vi "generate_tuning_spline.vi"(0 "Laser Power Q":T3, 11 "error in":errorcluster, 12 "Controls Cluster":T2 {"Initial Step Direction" items=["Negative", "Positive"]}, 13 "file path (dialog if empty)":path, 14 "Bounds":T1) -> (4 "Opt Data":cluster{dbl[], dbl[]}, 15 "error out":errorcluster)   [LabVIEW 2023]
uses:
  <vilib>/Utility/file.llb/Write Delimited Spreadsheet (DBL).vi
panel:
  in  "Cancel Optimisation":bool
  in  "stop":bool
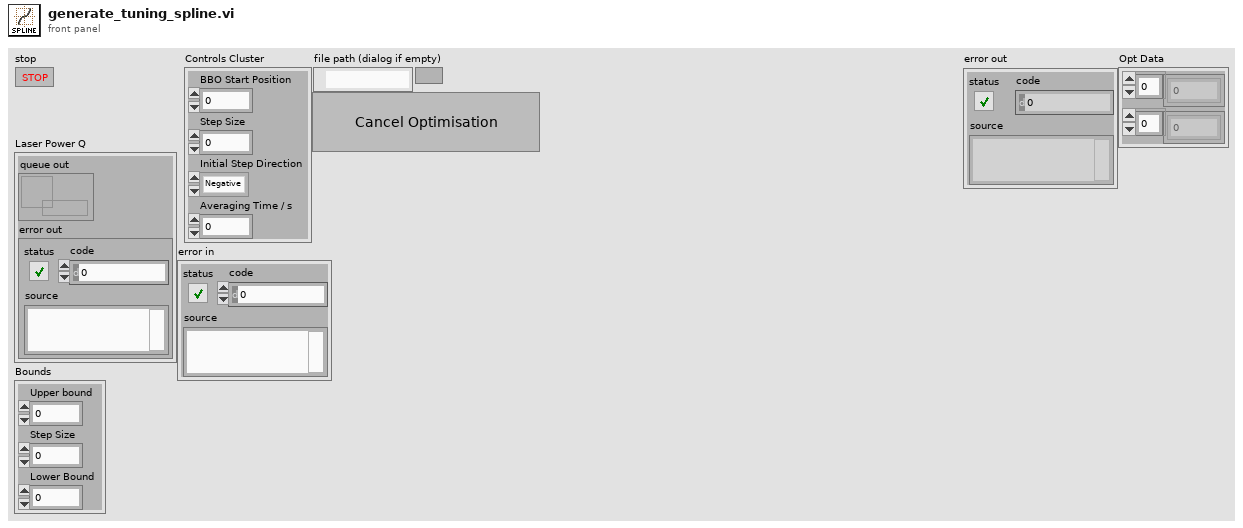
[diagram p1: front panel]
types:
  T1 = cluster{"Upper bound":dbl, "Step Size":dbl, "Lower Bound":dbl}
  T2 = cluster{"BBO Start Position":i32, "Step Size":i32, "Initial Step Direction":u16, "Averaging Time / s ":u32}
  T3 = cluster{"queue out":refnum<queue>, "error out":errorcluster}
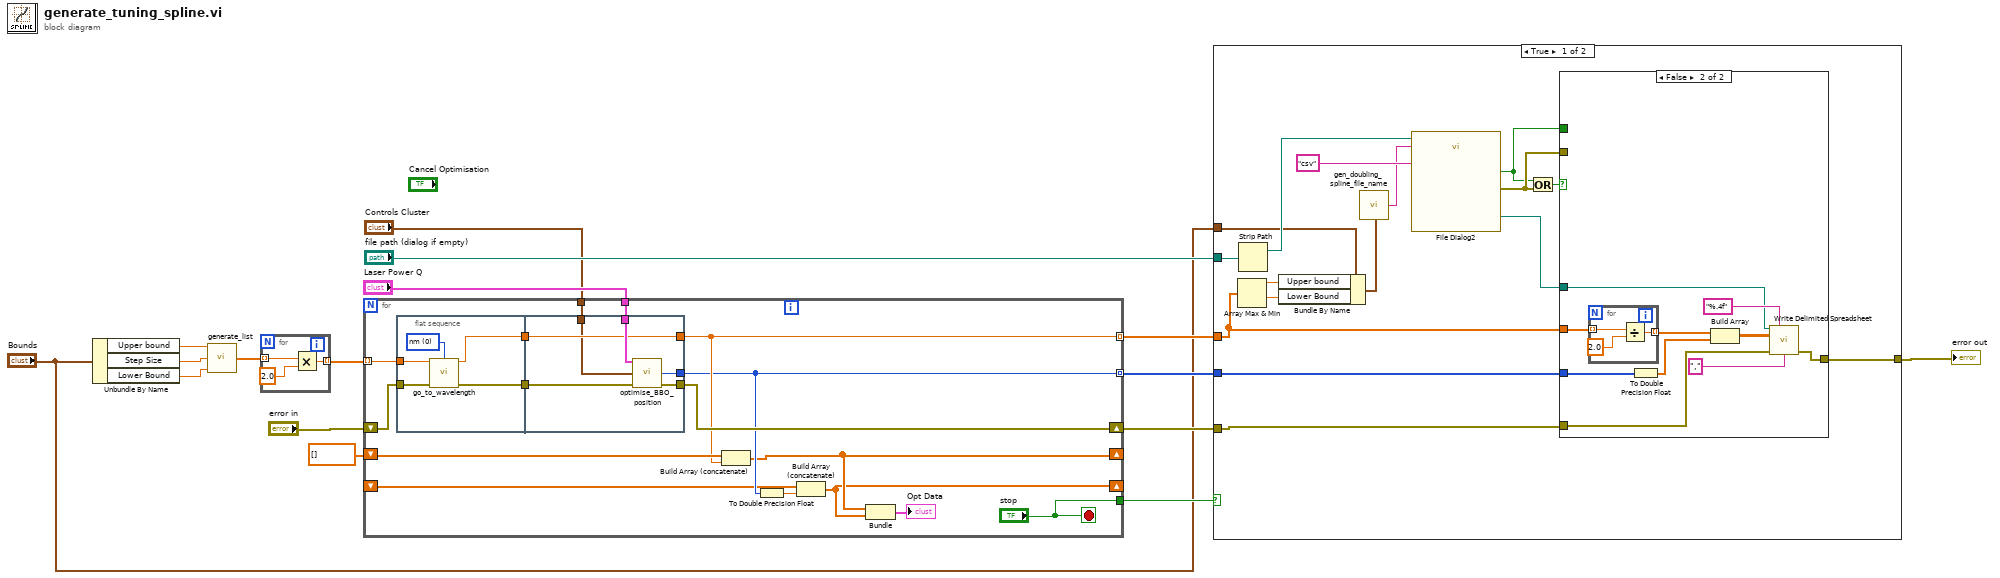
[diagram p0: block diagram]
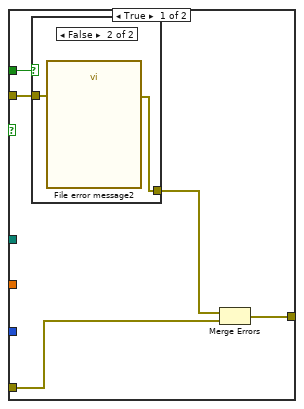
[diagram p2: hidden frame]
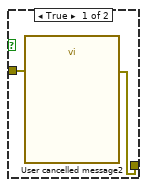
[diagram p3: hidden frame]
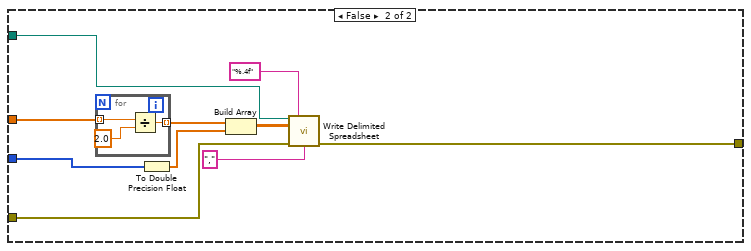
[diagram p4: hidden frame]
diagram:
  n1 = Unbundle By Name("Bounds") -> ("Upper bound"=w8:dbl, "Step Size"=w7:dbl, "Lower Bound"=w6:dbl)
  n2 = call "generate_list.vi"("Upper bound"=w8, "Step Size"=w7, "Lower Bound"=w6) -> ("Array"=w16:dbl[])  [unwired: 12 in]
  n3 = for {
    tunnel: w16 -> [w19] mode=indexing
    tunnel: [w17] -> w15 mode=indexing
    n4 = Multiply(x=w19, y=2.0) -> (x*y=w17:dbl)
  }
  n5 = for {
    tunnel: w15 -> [w35] mode=indexing
    shift-right: [w32] -> w10
    shift-left: "error in" -> [w34]
    tunnel: "Laser Power Q" -> [w31]
    tunnel: [w27] -> w11 mode=indexing
    tunnel: [w28] -> w12 mode=indexing
    shift-right: [w24] -> _
    shift-left: dbl[] [] -> [w29]
    shift-right: [w23] -> _
    shift-left: _ -> [w25]
    tunnel: "Controls Cluster" -> [w21]
    tunnel: ["stop"] -> w4
    stop <- "stop" stop-if-true
    n6 = flat-sequence {
      tunnel: w35 -> [w40]
      tunnel: w34 -> [w39]
      tunnel: [w37] -> w33
      tunnel: [w36] -> w30
      tunnel: [w44] -> w32
      tunnel: w33 -> [w46]
      tunnel: w31 -> [w45]
      tunnel: [w43] -> w27
      tunnel: w30 -> [w42]
      tunnel: [w42] -> w28
      tunnel: w21 -> [w41]
      frame #0 {
        w38 = u16 0 items=["nm", "cm-1"] ("Unit")
        n7 = call "go_to_wavelength.vi"("Set Laser Position"=w40, "Unit"=w38, "error in (no error)"=w39) -> ("Current Laser Position"=w36:dbl, "error out"=w37:errorcluster)  [unwired: 11 in]
      }
      frame #1 {
        n8 = call "optimise_BBO_position.vi"("Laser Power Q"=w45, "Controls Cluster"=w41, "error in (no error)"=w46) -> ("Optimised BBO crystal position"=w43:i32, "error out"=w44:errorcluster)  [unwired: 11 in]
      }
    }
    n9 = Build Array (concatenate)(w29, w28) -> (w24:dbl[])
    n10 = To Double Precision Float(number=w27) -> (double precision float=w26:dbl)
    n11 = Build Array (concatenate)(w25, w26) -> (w23:dbl[])
    n12 = Bundle(w24, w23) -> (→"Opt Data":cluster{dbl[], dbl[]})  [unwired: 1 in]
  }
  n13 = case shown="True" w4 {
    tunnel: w12 -> [w53 w94]
    tunnel: w11 -> [w56 w93]
    tunnel: w10 -> [w57 w89]
    tunnel: "file path (dialog if empty)" -> [w62 w86]
    tunnel: [w47 w85] -> w3
    tunnel: "Bounds" -> [w52 _]
    frame True {
      n14 = Array Max & Min(array=w53) -> (max value=w51:dbl, min value=w50:dbl)  [unwired: 2 out]
      n15 = Strip Path(path=w62) -> (stripped path=w54:path)  [unwired: 1 out]
      n16 = Bundle By Name(cluster=w52, "Upper bound"=w51, "Lower Bound"=w50) -> (w49:T1)
      n17 = call "gen_doubling_spline_file_name.vi"("output cluster"=w49) -> ("concatenated string"=w48:string)  [unwired: 14 in]
      n18 = call "File Dialog2"("start path"=w54, "default name"=w48, "pattern (all files)"="csv") -> ("selected path"=w59:path, "cancelled"=w60:bool, "error out"=w61:errorcluster)  [unwired: 9 in, 1 out]
      n19 = Or(x=w60, y=w61) -> (x .or. y?=w58:bool)
      n20 = case shown="False" w58 {
        tunnel: w59 -> [_ w73]
        tunnel: w60 -> [w67 _]
        tunnel: w61 -> [w66 _]
        tunnel: w57 -> [w63 w77]
        tunnel: w56 -> [_ w76]
        tunnel: w53 -> [_ w75]
        tunnel: [w64 w72] -> w47
        frame True {
          n21 = case shown="False" w67 {
            tunnel: w66 -> [w69 w71]
            tunnel: [w68 w70] -> w65
            frame True {
              n22 = call "User cancelled message2"("error in (no error)"=w69) -> ("error out"=w68:errorcluster)  [unwired: 9 in, 1 out]
            }
            frame False {
              n23 = call "File error message2"("error in (no error)"=w71) -> ("error out"=w70:errorcluster)  [unwired: 9 in, 1 out]
            }
          }
          n24 = Merge Errors(w65, w63) -> (w64:errorcluster)
        }
        frame False {
          n25 = for {
            tunnel: w75 -> [w84] mode=indexing
            tunnel: [w82] -> w81 mode=indexing
            n26 = Divide(x=w84, y=2.0) -> (x/y=w82:dbl)
          }
          n27 = To Double Precision Float(number=w76) -> (double precision float=w80:dbl[])
          n28 = Build Array(w81, w80) -> (w79:dbl[][])
          n29 = call-poly <vilib>:"Write Delimited Spreadsheet.vi"("file path (dialog if empty)"=w73, "format (%.3f)"="%.4f", "2D data"=w79, "error in (no error)"=w77, "delimiter (\\t)"="," ("delimiter (\\t)")) -> ("error out"=w72:errorcluster)  [unwired: 9 in, 1 out]
        }
      }
    }
    frame False {
      n30 = for {
        tunnel: w94 -> [w97] mode=indexing
        tunnel: [w95] -> w92 mode=indexing
        n31 = Divide(x=w97, y=2.0) -> (x/y=w95:dbl)
      }
      n32 = To Double Precision Float(number=w93) -> (double precision float=w91:dbl[])
      n33 = Build Array(w92, w91) -> (w90:dbl[][])
      n34 = call-poly <vilib>:"Write Delimited Spreadsheet.vi"("file path (dialog if empty)"=w86, "format (%.3f)"="%.4f", "2D data"=w90, "error in (no error)"=w89, "delimiter (\\t)"="," ("delimiter (\\t)")) -> ("error out"=w85:errorcluster)  [unwired: 9 in, 1 out]
    }
  }
  "error out" <- w3
